vi "Write HDF5.vi"(8 "error in (no error)":errorcluster, 10 "path":path, 11 "LVtoITX in":refnum<class "LVtoITX.lvclass">) -> (0 "error out":errorcluster, 3 "LVtoITX out":refnum<class "LVtoITX.lvclass">)   [LabVIEW 2016, in "LVtoITX.lvclass"]
uses:
  LVtoITX.lvclass
  <vilib>/addons/h5labview2/file/H5Fmode.ctl
  LVtoITX.lvclass/LVtoITX.ctl
  <vilib>/addons/h5labview2/base/lib_path.vi
  <vilib>/addons/h5labview2/base/H5Equery.vi
  <vilib>/addons/h5labview2/base/hid_t.ctl
  <vilib>/addons/h5labview2/dataset/H5Dwrite.llb/H5Dwrite.xnode
  <vilib>/addons/h5labview2/file/H5F.lvlib
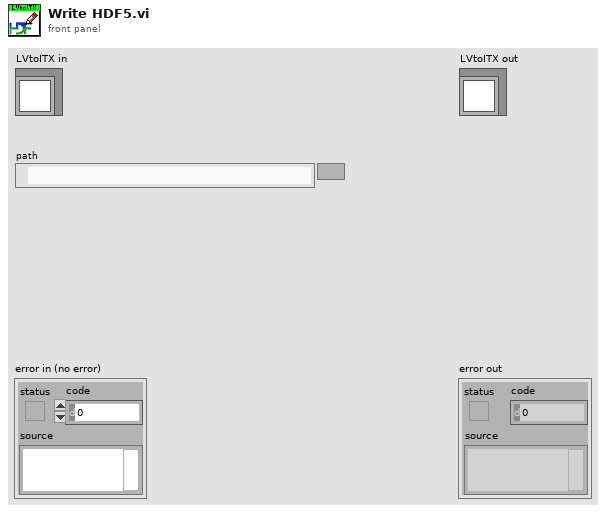
[diagram p1: front panel]
types:
  T1 = typedef "H5F.lvlib/H5Fmode.ctl" = enum16{"read-only", "read-write", "overwrite", "create new", "open or create"}
  T2 = typedef "hid_t.ctl" = i32
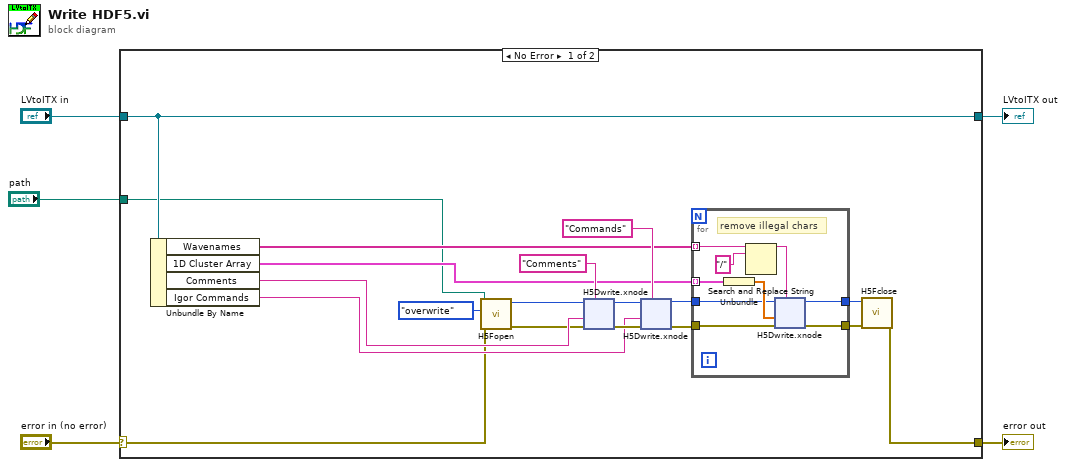
[diagram p0: block diagram]
diagram:
  n1 = case shown="No Error" "error in (no error)" {
    selector: "error in (no error)" -> [w7 w91]
    tunnel: [w17 w91] -> w2
    tunnel: [w16 w92] -> w3
    tunnel: "LVtoITX in" -> [w16 w92]
    tunnel: "path" -> [w6 _]
    frame No Error {
      n2 = Unbundle By Name(w16) -> ("Wavenames"=w15:string[], "1D Cluster Array"=w14:cluster{"array type (2D Dbl)":dbl[]}[], "Comments"=w13:string, "Igor Commands"=w12:string)
      n3 = call <vilib>:"H5Fopen.vi"("error in (no error)"=w7, "mode (read-only)"=H5Fmode."overwrite" ("mode"), "path"=w6) -> ("error out"=w8:errorcluster, "ref out"=w10:T2)  [unwired: 7 in]
      n4 = xnode "H5Dwrite.xnode"("dataset name"="Comments" ("attrib name"), "error in (no error)"=w8, "data"=w13, "ref in"=w10) -> ("error out"=w22:errorcluster, "ref out"=w21:T2)  [unwired: 3 in, 1 out]
      n5 = xnode "H5Dwrite.xnode"("dataset name"="Commands" ("attrib name"), "error in (no error)"=w22, "data"=w12, "ref in"=w21) -> ("error out"=w20:errorcluster, "ref out"=w18:T2)  [unwired: 3 in, 1 out]
      n6 = for {
        tunnel: w15 -> [w65] mode=indexing
        tunnel: w14 -> [w71] mode=indexing
        tunnel: w18 -> [w67]
        tunnel: [w66] -> w9
        tunnel: w20 -> [w68]
        tunnel: [w69] -> w11
        # "remove illegal chars"
        n7 = Unbundle(w71) -> ("array type (2D Dbl)"=w70:dbl[])
        n8 = Search and Replace String(input string=w65, search string="/") -> (result string=w64:string)  [unwired: 6 in, 3 out]
        n9 = xnode "H5Dwrite.xnode"("dataset name"=w64, "error in (no error)"=w68, "data"=w70, "ref in"=w67) -> ("error out"=w69:errorcluster, "ref out"=w66:T2)  [unwired: 3 in, 1 out]
      }
      n10 = call <vilib>:"H5Fclose.vi"("error in (no error)"=w11, "ref"=w9) -> ("error out"=w17:errorcluster)  [unwired: 9 in]
    }
    frame Error {
    }
  }
  "error out" <- w2
  "LVtoITX out" <- w3
